vi "Set 2D Field (Cartesian).vi"(2 "error in":T2, 4 "Z-Axis Field (T)":dbl format="%.3f", 6 "Z-Axis Communications Config":T1={"GPIB address"=22, "GPIB bus"=0, "connection ID"=refnum, "IP"="192.168.2.200", "Active Comm Interface"=0, "Serial Port"="", "Programmer Type"=0} {"Programmer Type" items=["Model 430", "Model 420"]; "Active Comm Interface" items=["TCP/IP (Model 430 Only)", "RS232", "IEEE488"]}, 7 "Y-Axis Field (T)":dbl format="%.3f", 8 "Y-Axis Communications Config":T1={"GPIB address"=22, "GPIB bus"=0, "connection ID"=refnum, "IP"="192.168.2.200", "Active Comm Interface"=0, "Serial Port"="", "Programmer Type"=0} {"Programmer Type" items=["Model 430", "Model 420"]; "Active Comm Interface" items=["TCP/IP (Model 430 Only)", "RS232", "IEEE488"]}) -> (0 "error out":T2, 1 "Within Limits?":bool)   [LabVIEW 2019]
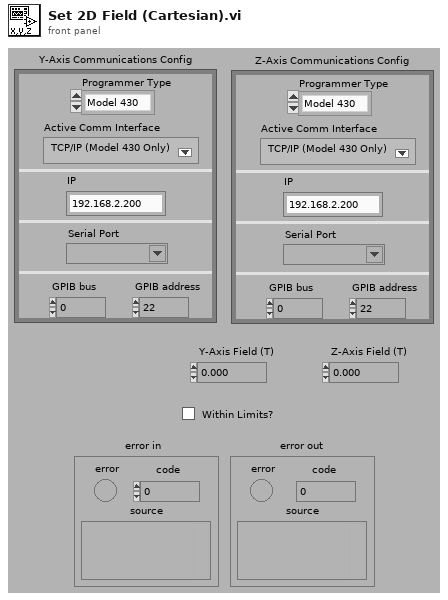
[diagram p1: front panel]
types:
  T1 = cluster{"GPIB address":i16, "GPIB bus":i16, "connection ID":refnum<k5>, "IP":string, "Active Comm Interface":u16, "Serial Port":refnum<visa-resource-name>, "Programmer Type":u16}
  T2 = cluster{"error":bool, "code":i32, "source":string}
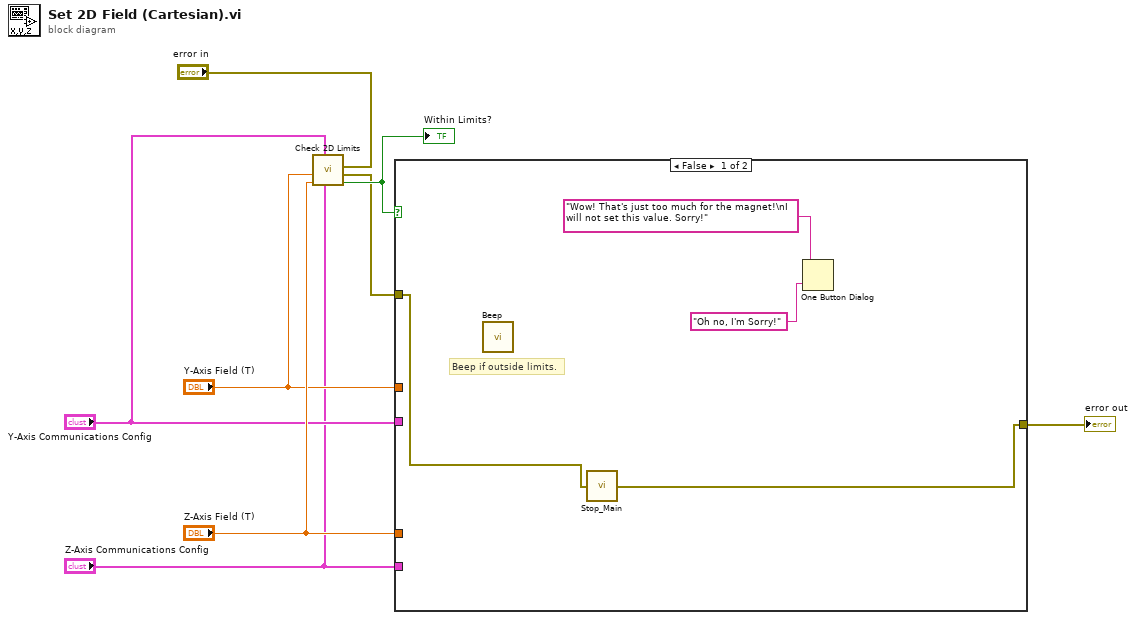
[diagram p0: block diagram]
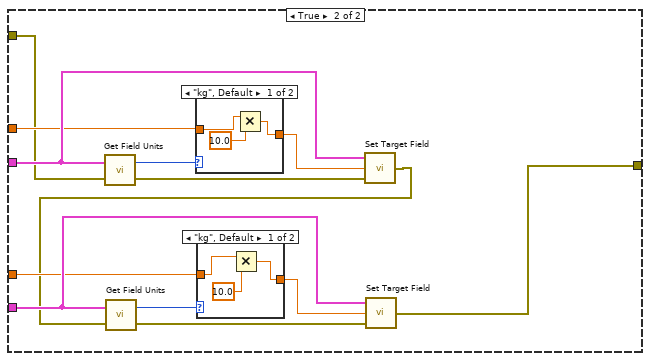
[diagram p2: hidden frame]
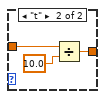
[diagram p3: hidden frame]
diagram:
  n1 = call "Check 2D Limits.vi"("error in"="error in", "Z-Axis Communications Config"="Z-Axis Communications Config", "Y-Axis Communications Config"="Y-Axis Communications Config", "Z-Axis Field (T)"="Z-Axis Field (T)", "Y-Axis Field (T)"="Y-Axis Field (T)") -> ("Within Limits?"=w6:bool, "error out"=w4:T2)  [unwired: 3 in]
  "Within Limits?" <- w6
  n2 = case shown="False" w6 {
    tunnel: "Y-Axis Communications Config" -> [_ w19]
    tunnel: "Y-Axis Field (T)" -> [_ w18]
    tunnel: "Z-Axis Field (T)" -> [_ w16]
    tunnel: "Z-Axis Communications Config" -> [_ w17]
    tunnel: w4 -> [w10 w13]
    tunnel: [w9 w14] -> w7
    frame False {
      # "Beep if outside limits."
      n3 = call <vilib>:"Beep.vi"() -> ()  [unwired: 12 in]
      n4 = call "Stop_Main.vi"("error in"=w10) -> ("error out"=w9:errorcluster)
      n5 = One Button Dialog(message="Wow! That's just too much for the magnet!\nI will not set this value. Sorry!", button name ("OK")="Oh no, I'm Sorry!") -> ()  [unwired: 1 out]
    }
    frame True {
      n6 = call "Get Field Units.vi"("error in"=w13, "Z-Axis Communications Config"=w19) -> ("error out"=w24:T2, "Field Units"=w25:enum16{"kg", "t"})
      n7 = case shown="\"kg\", Default" w25 {
        tunnel: [w33 w35] -> w23
        tunnel: w18 -> [w34 w35]
        frame "kg", Default {
          n8 = Multiply(x=w34, y=10.0) -> (x*y=w33:dbl)
        }
        frame "t" {
        }
      }
      n9 = call "Set Target Field.vi"("error in"=w24, "Target Field (kG)"=w23, "Communications Config"=w19) -> ("error out"=w15:T2)
      n10 = call "Get Field Units.vi"("error in"=w15, "Z-Axis Communications Config"=w17) -> ("error out"=w21:T2, "Field Units"=w22:enum16{"kg", "t"})
      n11 = case shown="\"kg\", Default" w22 {
        tunnel: [w27 w30] -> w20
        tunnel: w16 -> [w28 w29]
        frame "kg", Default {
          n12 = Multiply(x=w28, y=10.0) -> (x*y=w27:dbl)
        }
        frame "t" {
          n13 = Divide(x=w29, y=10.0) -> (x/y=w30:dbl)
        }
      }
      n14 = call "Set Target Field.vi"("error in"=w21, "Target Field (kG)"=w20, "Communications Config"=w17) -> ("error out"=w14:T2)
    }
  }
  "error out" <- w7
